vi "Contabilidad.vi"(8 "error in (no error)":errorcluster, 11 "User Interface in":refnum<class "User Interface.lvclass">) -> (0 "error out":errorcluster, 3 "User Interface out":refnum<class "User Interface.lvclass">)   [LabVIEW 2020, in "User Interface.lvlib" / "User Interface.lvclass"]
uses:
  User Interface.lvclass
  User Interface.lvclass/User Interface.ctl
panel:
  in  "End Time":timestamp
  in  "Start Time":timestamp
  in  "Cancel":bool
  in  "Request":bool
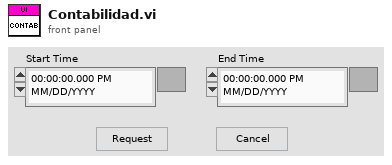
[diagram p1: front panel]
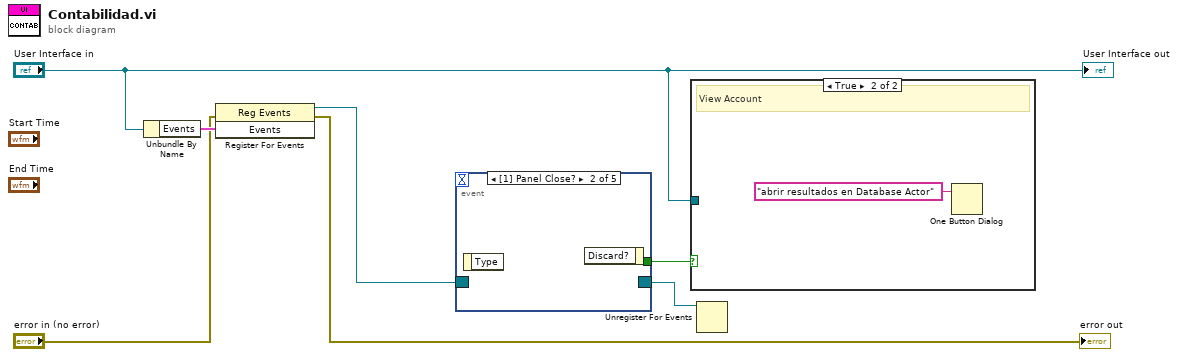
[diagram p0: block diagram]
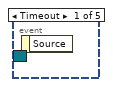
[diagram p2: hidden frame]
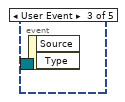
[diagram p3: hidden frame]
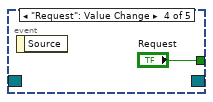
[diagram p4: hidden frame]
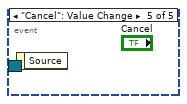
[diagram p5: hidden frame]
diagram:
  n1 = Unbundle By Name("User Interface in") -> ("Events"=w6:cluster{"Stop":refnum<user-event>})
  n2 = register-events(error in="error in (no error)", w6) -> (reference out=w3:refnum<event-registration>, error out=→"error out":errorcluster)  [unwired: 1 in]
  n3 = event shown="[1] Panel Close?" {
    selector: w3 -> [_ _ _ _ _]
    dyn-events: [_ _ _ _ _] -> w1
    timeout: _ -> [_ _ _ _ _]
    tunnel: [_ _ _ "Request" _] -> w7
    event Timeout {
      n4 = event-data() -> ()  [unwired: 1 in, 1 out]
    }
    event Panel Close? {
      n5 = event-data() -> ()  [unwired: 1 in, 1 out]
      n6 = event-data() -> ()  [unwired: 2 in, 1 out]
    }
    event User Event {
      n7 = event-data() -> ()  [unwired: 1 in, 2 out]
    }
    event "Request": Value Change {
      n8 = event-data() -> ()  [unwired: 1 in, 1 out]
    }
    event "Cancel": Value Change {
      n9 = event-data() -> ()  [unwired: 1 in, 1 out]
    }
  }
  n10 = case shown="True" w7 {
    tunnel: "User Interface in" -> [_ _]
    frame False {
    }
    frame True {
      # "View Account"
      n11 = One Button Dialog(message="abrir resultados en Database Actor") -> ()  [unwired: 1 in, 1 out]
    }
  }
  n12 = Unregister For Events(event registration refnum=w1) -> ()  [unwired: 1 in, 1 out]
  "User Interface out" <- "User Interface in"
